vi "Clear Dictionary.vi"(8 "error in (no error)":errorcluster, 11 "SMO.Dictionary in":refnum<class "SMO.Dictionary.lvclass">) -> (0 "error out":errorcluster, 3 "SMO.Dictionary out":refnum<class "SMO.Dictionary.lvclass">)   [LabVIEW 2013, in "SMO.Dictionary.lvlib" / "SMO.Dictionary.lvclass"]
uses:
  SMO.Dictionary.lvclass
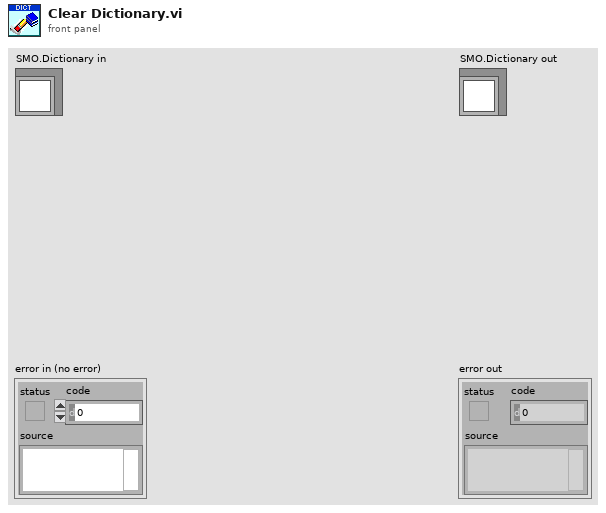
[diagram p1: front panel]
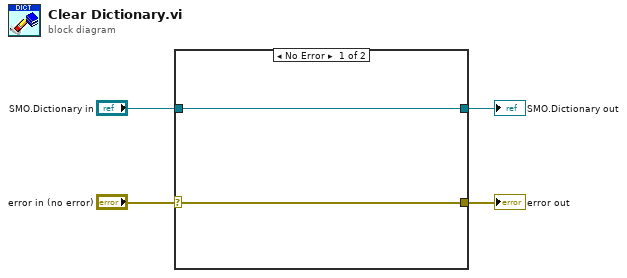
[diagram p0: block diagram]
diagram:
  n1 = case shown="No Error" "error in (no error)" {
    selector: "error in (no error)" -> [w5 w8]
    tunnel: [w5 w8] -> w3
    tunnel: [w6 w7] -> w1
    tunnel: "SMO.Dictionary in" -> [w6 w7]
    frame No Error {
    }
    frame Error {
    }
  }
  "error out" <- w3
  "SMO.Dictionary out" <- w1
